vi "Constant - Analog Input Channel Lookup Table.vi"() -> (2 "Analog Channel Lookup Table":i32[](array[numeric])=[1, 3, 7, 15, 31, 63, 127, 255, 511, 1023, 2047, 4095, 8191, 16383, 32767, 65535])   [LabVIEW 2021]
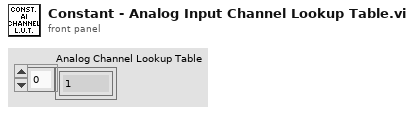
[diagram p1: front panel]
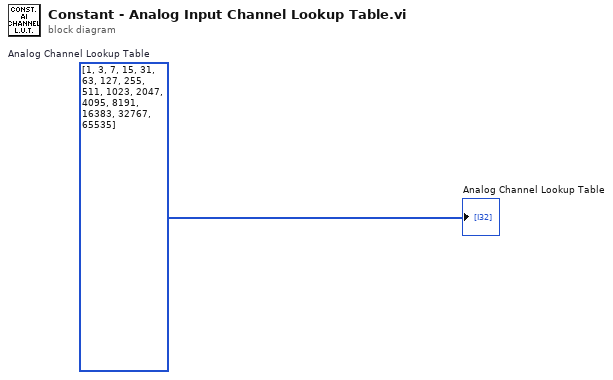
[diagram p0: block diagram]
diagram:
  w1 = i32[] [1, 3, 7, 15, 31, 63, 127, 255, 511, 1023, 2047, 4095, 8191, 16383, 32767, 65535]  # Analog Channel Lookup Table
  "Analog Channel Lookup Table" <- w1
